vi "TURCK GUI TestPanel AI.vi"() -> ()   [LabVIEW 2021]
doc: "Example for reading Values from TBEN-S2-4AI module from Turck"
uses:
  KH TURCK ETHERNETIP TDefCluster TBEN-S2-4AI Input Values.ctl
  KH EthernetIP 17.19/KH_EthernetIP_Globals.vi
panel:
  out "TBEN-S2-4AI Input Values":T1
  out "upper Limit CH3":bool caption="upper Limit"
  out "Analog Input 3":i16(knob) scale=15000.0..65535.0
  out "upper Limit CH2":bool caption="upper Limit"
  out "Analog Input 2":i16(knob) scale=15000.0..65535.0
  out "upper Limit CH1":bool caption="upper Limit"
  out "Analog Input 1":i16(knob) scale=15000.0..65535.0
  out "error out":errorcluster
  out "upper Limit CH0":bool caption="upper Limit"
  out "Analog Input 0":i16(knob) scale=15000.0..65535.0
  in  "Exit":bool
  # "- Before starting the VI your PC has to be in the same subnet as the modules"
  # "Kirschenhofer Maschinen GmbH\nRömerstraße 35, 89278 Nersingen-Straß\ninfo@kirschenhofer-gmbh.de"
  # "Wire Break"
  # "upper limit"
  # "Overflow"
  # "Underflow"
  # "CJC Wire Break"
  # "Overcurrent (RTD)"
  # "Overcurrent supply VAUX1"
  # "Lower limit value underrun"
  # "Ch0"
  # "Ch1"
  # "Ch2"
  # "Ch3"
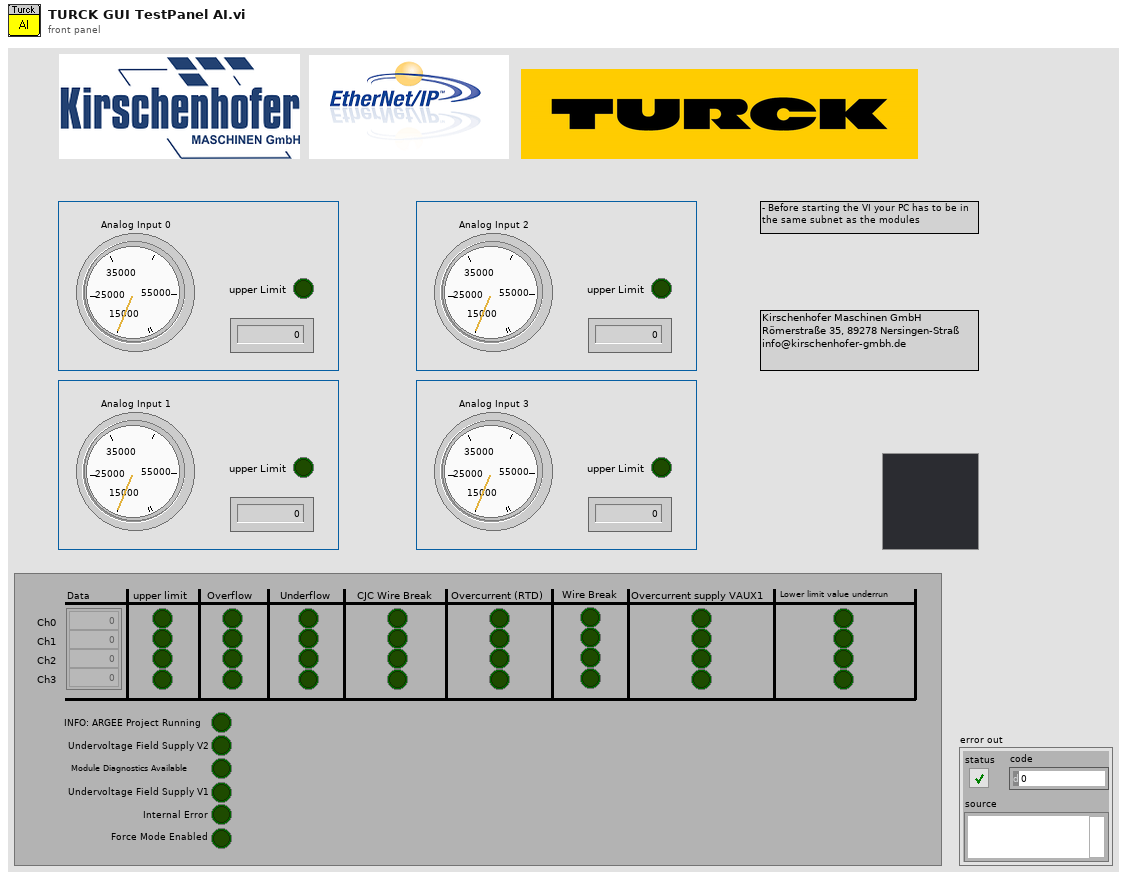
[diagram p1: front panel]
types:
  T1 = typedef "KH TURCK ETHERNETIP TDefCluster TBEN-S2-4AI Input Values.ctl" = cluster{"Data":i16[], "upper Limit CH0":bool, "upper Limit CH1":bool, "upper Limit CH2":bool, "upper Limit CH3":bool, "Overflow CH0":bool, "Overflow CH1":bool, "Overflow CH2":bool, "Overflow CH3":bool, "Underflow CH0":bool, "Underflow CH1":bool, "Underflow CH2":bool, "Underflow CH3":bool, "CJC Wire Break CH0":bool, "CJC Wire Break CH1":bool, "CJC Wire Break CH2":bool, "CJC Wire Break CH3":bool, "Overcurrent (RTD) CH0":bool, "Overcurrent (RTD) CH1":bool, "Overcurrent (RTD) CH2":bool, "Overcurrent (RTD) CH3":bool, "Wire Break CH0":bool, "Wire Break CH1":bool, "Wire Break CH2":bool, "Wire Break CH3":bool, "Overcurrent supply VAUX1 CH0":bool, "Overcurrent supply VAUX1 CH1":bool, "Overcurrent supply VAUX1 CH2":bool, "Overcurrent supply VAUX1 CH3":bool, "Lower limit value underrun CH0":bool, "Lower limit value underrun CH1":bool, "Lower limit value underrun CH2":bool, "Lower limit value underrun CH3":bool, "Module Diagnostics Available":bool, "INFO: ARGEE Project Running":bool, "Undervoltage Field Supply V2":bool, "Undervoltage Field Supply V1":bool, "Internal Error":bool, "Force Mode Enabled":bool}
  T2 = cluster{"ItemCount":u16, "AdressItem":cluster{"TypeID":u16, "Length":u16, "Data":cluster{"ConnectionIdentifier":u32, "SequenceNumber":u32}}, "DataItem":cluster{"TypeID":u16, "Length":u16, "Data":u8[], "Sequence Count":u16}}
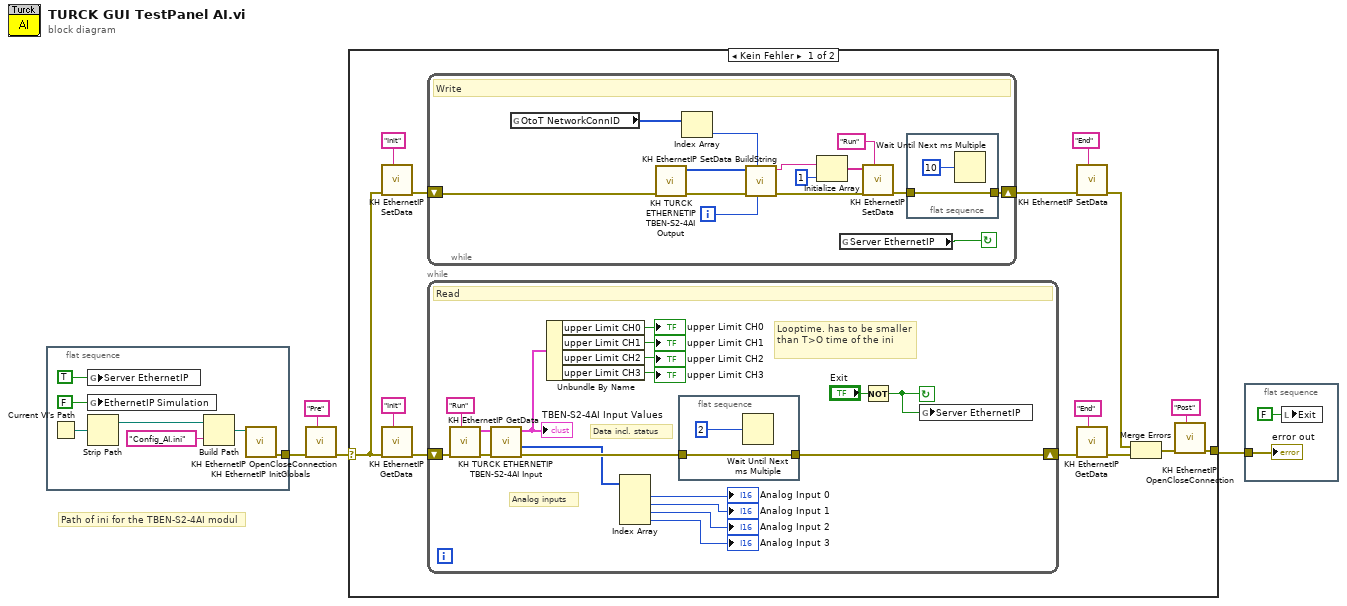
[diagram p0: block diagram]
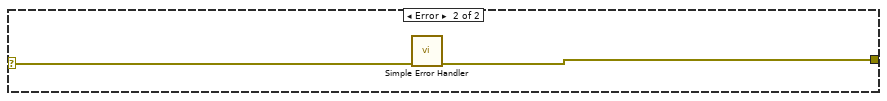
[diagram p2: hidden frame]
diagram:
  # "Path of ini for the TBEN-S2-4AI modul"
  n1 = flat-sequence {
    tunnel: [w11] -> w2
    frame #0 {
      n2 = Current VI's Path() -> (path=w7:path)
      n3 = global write "KH_EthernetIP_Globals.vi" "Server EthernetIP"(TRUE ("Server EthernetIP")) -> ()
      n4 = global write "KH_EthernetIP_Globals.vi" "EthernetIP Simulation"(FALSE ("EthernetIP Simulation")) -> ()
      n5 = Strip Path(path=w7) -> (stripped path=w9:path)  [unwired: 1 out]
      n6 = Build Path(base path=w9, name or relative path="Config_AI.ini") -> (appended path=w5:path)
      n7 = call "KH EthernetIP InitGlobals.vi"("Config File"=w5) -> ("err out"=w11:errorcluster)  [unwired: 10 in]
    }
  }
  n8 = call "KH EthernetIP OpenCloseConnection.vi"("Function"="Pre", "error in"=w2) -> ("error out"=w1:errorcluster)  [unwired: 9 in]
  n9 = case shown="Kein Fehler" w1 {
    selector: w1 -> [w12 w63]
    tunnel: [w13 w62] -> w3
    frame No Error {
      n10 = call "KH EthernetIP SetData.vi"("Function"="Init", "error in"=w12) -> ("error out"=w24:errorcluster)  [unwired: 7 in, 2 out]
      n11 = call "KH EthernetIP GetData.vi"("Function"="Init", "error in"=w12) -> ("error out"=w14:errorcluster)  [unwired: 8 in, 1 out]
      n12 = while {
        shift-right: [w37] -> w23
        shift-left: w24 -> [w29]
        i -> [w33]
        stop <- w36 continue-if-true
        # "Write"
        n13 = global read "KH_EthernetIP_Globals.vi" "OtoT NetworkConnID"() -> (w26:u32[])
        n14 = call "KH TURCK ETHERNETIP TBEN-S2-4AI Output.vi"("error in"=w29) -> ("error out"=w34:errorcluster, "Output Data"=w35:u8[])  [unwired: 9 in]
        n15 = Index Array(array=w26) -> (element=w27:u32)  [unwired: 1 in]
        n16 = call "KH EthernetIP SetData BuildString.vi"("LoopIndex"=w33, "OtoT NetworkConnID"=w27, "error in"=w34, "Output Data"=w35) -> ("error out"=w28:errorcluster, "DataString"=w32:string)  [unwired: 6 in]
        n17 = Initialize Array(w32, 1 ("dimension size")) -> (w30:string[])
        n18 = global read "KH_EthernetIP_Globals.vi" "Server EthernetIP"() -> (w36:bool)
        n19 = call "KH EthernetIP SetData.vi"("Function"="Run", "error in"=w28, "Data Strings"=w30) -> ("error out"=w38:errorcluster)  [unwired: 6 in, 2 out]
        n20 = flat-sequence {
          tunnel: w38 -> [w40]
          tunnel: [w40] -> w37
          frame #0 {
            n21 = Wait Until Next ms Multiple(millisecond multiple=u32 10) -> ()  [unwired: 1 out]
          }
        }
      }
      n22 = while {
        shift-right: [w57] -> w16
        shift-left: w14 -> [w59]
        stop <- w52 continue-if-true
        # "Looptime. has to be smaller than T>O time of the ini"
        # "Data incl. status"
        # "Analog inputs"
        # "Read"
        n23 = call "KH EthernetIP GetData.vi"("Function"="Run", "error in"=w59) -> ("error out"=w56:errorcluster, "Response Data"=w54:T2)  [unwired: 8 in]
        n24 = call "KH TURCK ETHERNETIP TBEN-S2-4AI Input.vi"("error in"=w56, "Response Data"=w54) -> ("error out"=w55:errorcluster, "DataAI"=w49:i16[], "TBEN-S2-4AI Input Values"=w44:T1)  [unwired: 7 in]
        "TBEN-S2-4AI Input Values" <- w44
        n25 = Unbundle By Name(w44) -> ("upper Limit CH0"=→"upper Limit CH0":bool, "upper Limit CH1"=→"upper Limit CH1":bool, "upper Limit CH2"=→"upper Limit CH2":bool, "upper Limit CH3"=→"upper Limit CH3":bool)
        n26 = Index Array(array=w49) -> (element #1=→"Analog Input 0":i16, element #2=→"Analog Input 1":i16, element #3=→"Analog Input 2":i16, element #4=→"Analog Input 3":i16)  [unwired: 4 in]
        n27 = flat-sequence {
          tunnel: w55 -> [w60]
          tunnel: [w60] -> w57
          frame #0 {
            n28 = Wait Until Next ms Multiple(millisecond multiple=u32 2) -> ()  [unwired: 1 out]
          }
        }
        n29 = Not(x="Exit") -> (.not. x?=w52:bool)
        n30 = global write "KH_EthernetIP_Globals.vi" "Server EthernetIP"(w52) -> ()
      }
      n31 = call "KH EthernetIP SetData.vi"("Function"="End", "error in"=w23) -> ("error out"=w19:errorcluster)  [unwired: 7 in, 2 out]
      n32 = call "KH EthernetIP GetData.vi"("Function"="End", "error in"=w16) -> ("error out"=w21:errorcluster)  [unwired: 8 in, 1 out]
      n33 = Merge Errors(w19, w21) -> (w20:errorcluster)
      n34 = call "KH EthernetIP OpenCloseConnection.vi"("Function"="Post", "error in"=w20) -> ("error out"=w13:errorcluster)  [unwired: 9 in]
    }
    frame Error {
      n35 = call <vilib>:"Simple Error Handler.vi"("error in (no error)"=w63) -> ("error out"=w62:errorcluster)  [unwired: 4 in, 4 out]
    }
  }
  n36 = flat-sequence {
    tunnel: w3 -> [w64]
    frame #0 {
      n37 = local write "Exit"(FALSE ("Exit")) -> ()
      "error out" <- w64
    }
  }
